vi "CIPC L2Enet FIFO.vi"() -> (3 "CIF_CIPC_L2Enet.lvclass":refnum<class "CIF_CIPC_L2Enet.lvclass">)   [LabVIEW 2021, in "CIF_CIPC_L2Enet.lvclass"]
uses:
  CIF_CIPC_L2Enet.lvclass
  CIF_CIPC_L2Enet.lvclass/CIF_CIPC_L2Enet.ctl
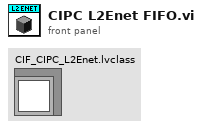
[diagram p1: front panel]
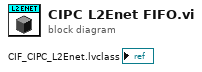
[diagram p0: block diagram]
diagram:
